vi "注册设备.vi"(11 "注册名称":string) -> ()   [LabVIEW 2018]
panel:
  in  "更新名称":bool
  in  "注册":bool
  out "设备GUID":string
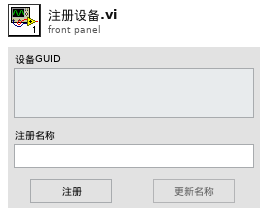
[diagram p1: front panel]
types:
  T1 = enum8{"Enabled", "Disabled", "Disabled and Grayed Out"}
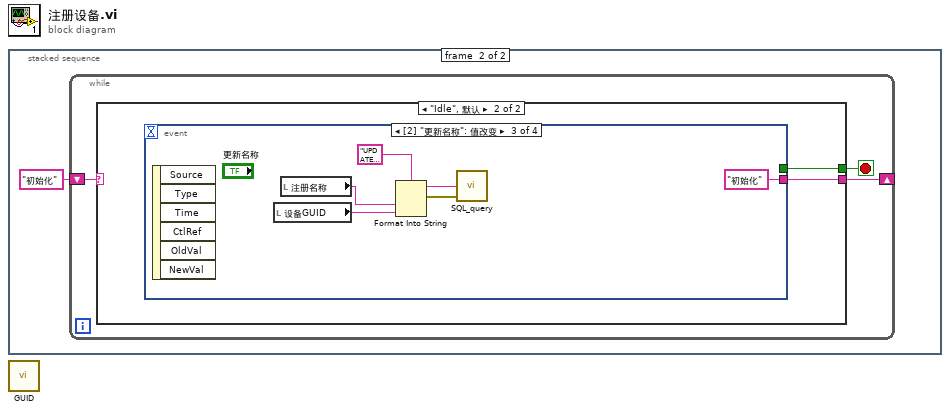
[diagram p0: block diagram]
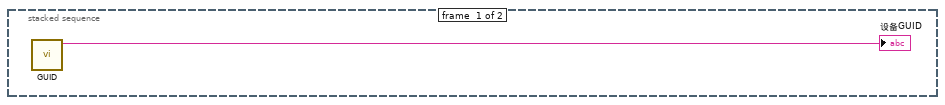
[diagram p2: hidden frame]
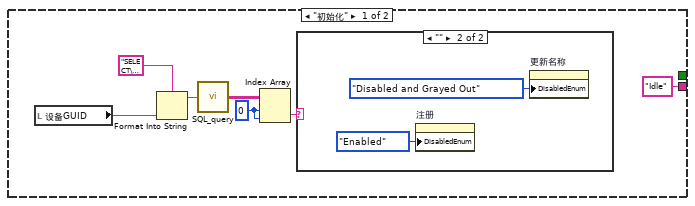
[diagram p3: hidden frame]
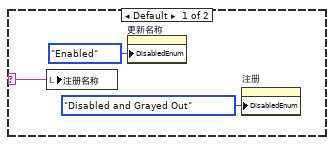
[diagram p4: hidden frame]
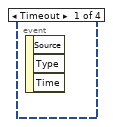
[diagram p5: hidden frame]
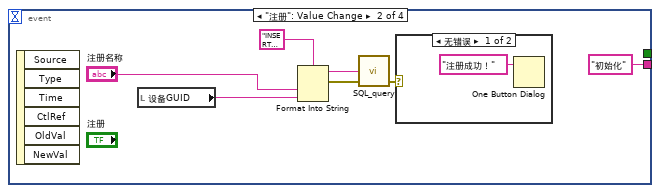
[diagram p6: hidden frame]
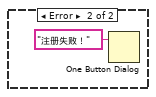
[diagram p7: hidden frame]
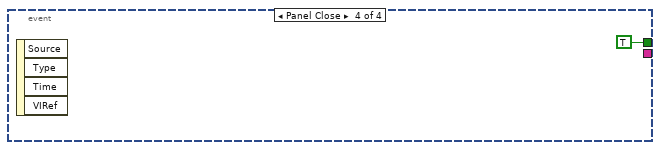
[diagram p8: hidden frame]
diagram:
  n1 = stacked-sequence {
    frame #0 {
      n2 = call "GUID.vi"() -> ("trimmed string"=→"设备GUID":string)  [unwired: 11 in]
    }
    frame #1 {
      n3 = while {
        shift-right: [w4] -> _
        shift-left: "初始化" -> [w5]
        stop <- w3 stop-if-true
        n4 = case shown="\"Idle\", 默认" w5 {
          tunnel: ["Idle" w19] -> w4
          tunnel: [_ w18] -> w3
          frame "初始化" {
            w9 = 0 ("索引 (行)")
            n5 = local read "设备GUID"() -> (w7:string)
            n6 = Format Into String(format string="SELECT\ndbo.Device.DEVICE_NAME\nFROM\ndbo.Device\nWHERE\ndbo.Device.DEVICE_PC_ID = '%s'\n", w7) -> (resulting string=w12:string)  [unwired: 2 in, 1 out]
            n7 = call "SQL_query.vi"("SQL query"=w12) -> ("data"=w11:string[][])  [unwired: 3 in, 1 out]
            n8 = Index Array(array=w11, index (row)=w9, index (col)=w9) -> (element=w10:string)
            n9 = case shown="\"\"" w10 {
              selector: w10 -> [w15 _]
              frame Default {
                n10 = local write "注册名称"(w15) -> ()
                n11 = property on="更新名称" class="Bool"("DisabledEnum"=T1."Enabled" ("禁用")) -> ()  [unwired: 2 in, 2 out]
                n12 = property on="注册" class="Bool"("DisabledEnum"=T1."Disabled and Grayed Out" ("禁用")) -> ()  [unwired: 2 in, 2 out]
              }
              frame "" {
                n13 = property on="注册" class="Bool"("DisabledEnum"=T1."Enabled" ("禁用")) -> ()  [unwired: 2 in, 2 out]
                n14 = property on="更新名称" class="Bool"("DisabledEnum"=T1."Disabled and Grayed Out" ("禁用")) -> ()  [unwired: 2 in, 2 out]
              }
            }
          }
          frame "Idle", Default {
            n15 = event shown="[2] \"更新名称\": 值改变" {
              selector: _ -> [_ _ _ _]
              dyn-events: _ -> [_ _ _ _]
              timeout: _ -> [_ _ _ _]
              tunnel: [_ "初始化" "初始化" _] -> w19
              tunnel: [_ _ _ TRUE] -> w18
              event Timeout {
                n16 = event-data() -> ()  [unwired: 1 in, 3 out]
              }
              event "注册": Value Change {
                n17 = event-data() -> ()  [unwired: 1 in, 6 out]
                n18 = local read "设备GUID"() -> (w23:string)
                n19 = Format Into String(format string="INSERT INTO dbo.Device ( Device.DEVICE_NAME,Device.DEVICE_PC_ID )\nVALUES\n\t(\n\t\tN'%s',\n\t'%s' \n\t)", "注册名称", w23) -> (resulting string=w25:string, error out=w24:errorcluster)  [unwired: 2 in]
                n20 = call "SQL_query.vi"("error in (no error)"=w24, "SQL query"=w25) -> ("error out"=w20:errorcluster)  [unwired: 2 in, 1 out]
                n21 = case shown="无错误" w20 {
                  frame No Error {
                    n22 = One Button Dialog(message="注册成功！" ("消息")) -> ()  [unwired: 1 in, 1 out]
                  }
                  frame Error {
                    n23 = One Button Dialog(message="注册失败！" ("消息")) -> ()  [unwired: 1 in, 1 out]
                  }
                }
              }
              event "更新名称": Value Change {
                n24 = event-data() -> ()  [unwired: 1 in, 6 out]
                n25 = local read "设备GUID"() -> (w31:string)
                n26 = local read "注册名称"() -> (w30:string)
                n27 = Format Into String(format string="UPDATE [dbo].[Device] SET [DEVICE_NAME] = N'%s' WHERE [DEVICE_PC_ID] = '%s'", w30, w31) -> (resulting string=w34:string, error out=w33:errorcluster)  [unwired: 2 in]
                n28 = call "SQL_query.vi"("error in (no error)"=w33, "SQL query"=w34) -> ()  [unwired: 2 in, 2 out]
              }
              event Panel Close {
                n29 = event-data() -> ()  [unwired: 1 in, 4 out]
              }
            }
          }
        }
      }
    }
  }
  n30 = call "GUID.vi"() -> ()  [unwired: 11 in, 1 out]
